vi "Custom_NAND.vi"(8 "Input B":bool, 11 "Input A":bool) -> (3 "Output":bool)   [LabVIEW 2026]
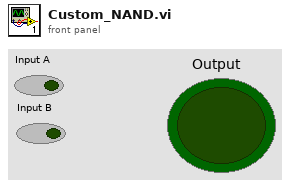
[diagram p1: front panel]
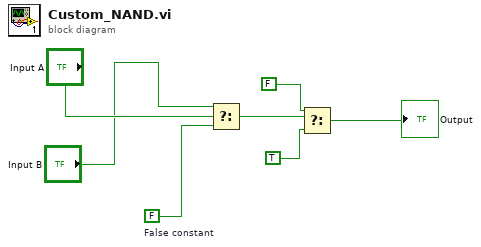
[diagram p0: block diagram]
diagram:
  w6 = FALSE  # False constant
  n1 = Select(t="Input B", s="Input A", f=w6) -> (s? t:f=w1:bool)
  n2 = Select(t=FALSE, s=w1, f=TRUE) -> (s? t:f=→"Output":bool)
